vi "Write color.vi"(8 "error in (no error)":errorcluster, 10 "color":u32, 11 "Component-B in":refnum<class "Component-B.lvclass">) -> (0 "error out":errorcluster, 3 "Component-B out":refnum<class "Component-B.lvclass">)   [LabVIEW 2018, in "Component-B.lvclass"]
uses:
  Component-B.lvclass
  Component-B.lvclass/Component-B.ctl
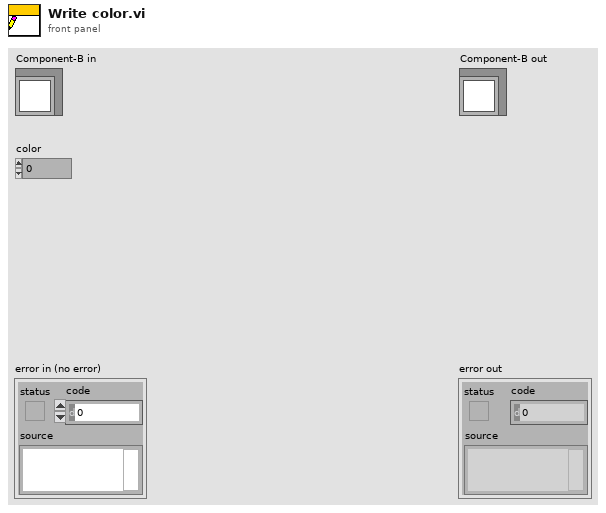
[diagram p1: front panel]
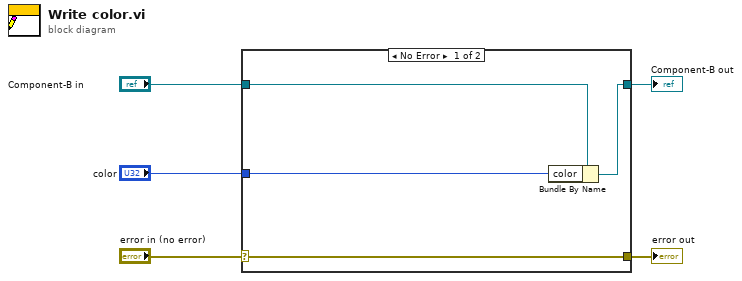
[diagram p0: block diagram]
diagram:
  n1 = case shown="No Error" "error in (no error)" {
    selector: "error in (no error)" -> [w9 w10]
    tunnel: [w9 w10] -> w4
    tunnel: [w7 w11] -> w2
    tunnel: "Component-B in" -> [w8 w11]
    tunnel: "color" -> [w6 _]
    frame No Error {
      n2 = Bundle By Name(cluster=w8, "color"=w6) -> (w7:refnum<class "Component-B.lvclass">)
    }
    frame Error {
    }
  }
  "error out" <- w4
  "Component-B out" <- w2
